vi "Configure Revert Worker.vi"() -> ()   [LabVIEW 2013, in "LVH-Revert.lvlib"]
uses:
  <vilib>/LabVIEW Hacker/Revert/LVH-Revert.lvlib
  <vilib>/Utility/config.llb/Read Key (String).vi
  <vilib>/Utility/config.llb/Read Key (Path).vi
  <vilib>/Utility/config.llb/Write Key (String).vi
  <vilib>/Utility/config.llb/Write Key (Path).vi
  <vilib>/Utility/config.llb/NI_LVConfig.lvlib
panel:
  in  "Archive Directory":path
  in  "Cancel Button":bool
  in  "Save Button":bool
  in  "Output Directory":path
  in  "Backsave Directory":path
  in  "Unzip Directory":path
  in  "Source Directory":path
  in  "Job Done Queue Name":string
  in  "Jobs Queue Name":string
  in  "AWS Account Number":string
  in  "AWS Secret Key":string
  in  "AWS Access Key ID":string
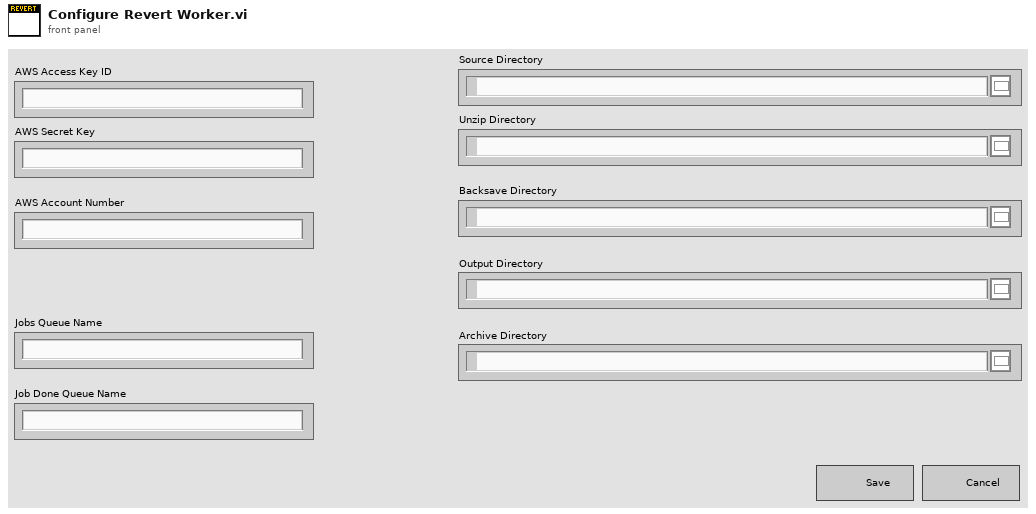
[diagram p1: front panel]
types:
  T1 = typedef "NI_LVConfig.lvlib/Config Data RefNum.ctl" = refnum<k1>
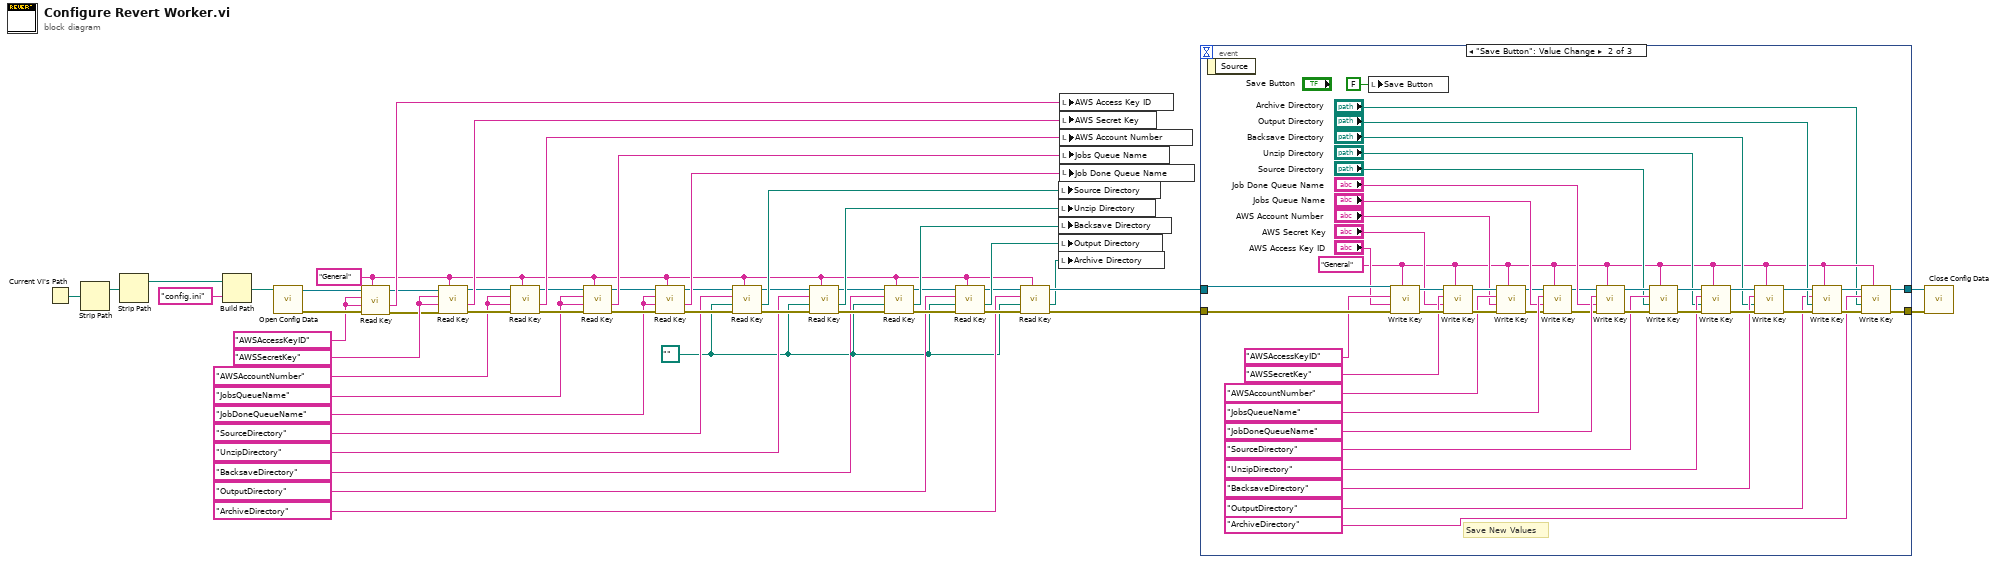
[diagram p0: block diagram]
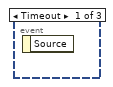
[diagram p2: hidden frame]
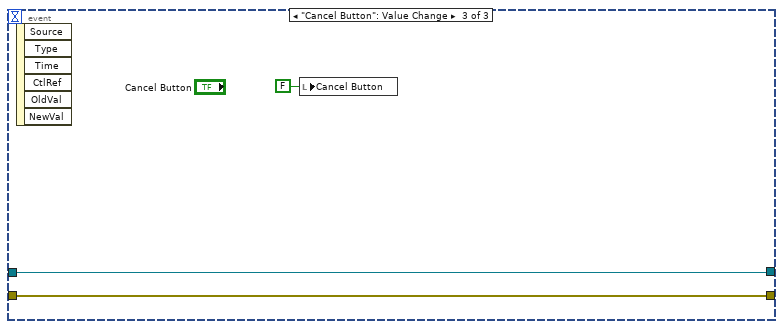
[diagram p3: hidden frame]
diagram:
  w2 = path "" ("Unzip Directory")
  w30 = "JobDoneQueueName"
  w32 = "JobsQueueName"
  w34 = "AWSAccountNumber"
  w36 = "AWSSecretKey"
  w38 = "AWSAccessKeyID"
  w4 = "General" ("section")
  n1 = Current VI's Path() -> (path=w51:path)
  n2 = Strip Path(path=w51) -> (stripped path=w50:path)  [unwired: 1 out]
  n3 = Strip Path(path=w50) -> (stripped path=w49:path)  [unwired: 1 out]
  n4 = Build Path(base path=w49, name or relative path="config.ini") -> (appended path=w47:path)
  n5 = call <vilib>:"Open Config Data.vi"("configuration file path"=w47) -> ("error out"=w46:errorcluster, "refnum"=w13:T1)  [unwired: 8 in, 1 out]
  n6 = call-poly <vilib>:"Read Key.vi"("section"=w4, "error in (no error)"=w46, "default value"=w38, "key"=w38, "refnum"=w13) -> ("error out"=w14:errorcluster, "value"=w37:string, "refnum out"=w12:T1)  [unwired: 3 in, 1 out]
  n7 = call-poly <vilib>:"Read Key.vi"("section"=w4, "error in (no error)"=w14, "default value"=w36, "key"=w36, "refnum"=w12) -> ("error out"=w45:errorcluster, "value"=w35:string, "refnum out"=w21:T1)  [unwired: 3 in, 1 out]
  n8 = call-poly <vilib>:"Read Key.vi"("section"=w4, "error in (no error)"=w45, "default value"=w34, "key"=w34, "refnum"=w21) -> ("error out"=w44:errorcluster, "value"=w33:string, "refnum out"=w20:T1)  [unwired: 3 in, 1 out]
  n9 = call-poly <vilib>:"Read Key.vi"("section"=w4, "error in (no error)"=w44, "default value"=w32, "key"=w32, "refnum"=w20) -> ("error out"=w43:errorcluster, "value"=w31:string, "refnum out"=w19:T1)  [unwired: 3 in, 1 out]
  n10 = call-poly <vilib>:"Read Key.vi"("section"=w4, "error in (no error)"=w43, "default value"=w30, "key"=w30, "refnum"=w19) -> ("error out"=w42:errorcluster, "value"=w29:string, "refnum out"=w18:T1)  [unwired: 3 in, 1 out]
  n11 = call-poly <vilib>:"Read Key.vi"("section"=w4, "error in (no error)"=w42, "default value"=w2, "key"="SourceDirectory", "refnum"=w18) -> ("error out"=w41:errorcluster, "value"=w27:path, "refnum out"=w17:T1)  [unwired: 3 in, 1 out]
  n12 = call-poly <vilib>:"Read Key.vi"("section"=w4, "error in (no error)"=w41, "default value"=w2, "key"="UnzipDirectory", "refnum"=w17) -> ("error out"=w40:errorcluster, "value"=w25:path, "refnum out"=w16:T1)  [unwired: 3 in, 1 out]
  n13 = call-poly <vilib>:"Read Key.vi"("section"=w4, "error in (no error)"=w40, "default value"=w2, "key"="BacksaveDirectory", "refnum"=w16) -> ("error out"=w39:errorcluster, "value"=w23:path, "refnum out"=w15:T1)  [unwired: 3 in, 1 out]
  n14 = call-poly <vilib>:"Read Key.vi"("section"=w4, "error in (no error)"=w39, "default value"=w2, "key"="OutputDirectory", "refnum"=w15) -> ("error out"=w8:errorcluster, "value"=w22:path, "refnum out"=w6:T1)  [unwired: 3 in, 1 out]
  n15 = call-poly <vilib>:"Read Key.vi"("section"=w4, "error in (no error)"=w8, "default value"=w2, "key"="ArchiveDirectory", "refnum"=w6) -> ("error out"=w7:errorcluster, "value"=w1:path, "refnum out"=w5:T1)  [unwired: 3 in, 1 out]
  n16 = local write "Source Directory"(w27) -> ()
  n17 = local write "Unzip Directory"(w25) -> ()
  n18 = local write "Backsave Directory"(w23) -> ()
  n19 = local write "Output Directory"(w22) -> ()
  n20 = local write "Archive Directory"(w1) -> ()
  n21 = local write "AWS Access Key ID"(w37) -> ()
  n22 = local write "AWS Secret Key"(w35) -> ()
  n23 = local write "AWS Account Number"(w33) -> ()
  n24 = local write "Jobs Queue Name"(w31) -> ()
  n25 = local write "Job Done Queue Name"(w29) -> ()
  n26 = event shown="[1] \"Save Button\": Value Change" {
    selector: _ -> [_ _ _]
    dyn-events: _ -> [_ _ _]
    timeout: _ -> [_ _ _]
    tunnel: w7 -> [_ w94 w97]
    tunnel: w5 -> [_ w93 w96]
    tunnel: [_ w55 w97] -> w10
    tunnel: [_ w56 w96] -> w9
    event Timeout {
      n27 = event-data() -> ()  [unwired: 1 in, 1 out]
    }
    event "Save Button": Value Change {
      w54 = "General" ("section")
      # "Save New Values"
      n28 = event-data() -> ()  [unwired: 1 in, 1 out]
      n29 = local write "Save Button"(FALSE ("Save Button")) -> ()
      n30 = call-poly <vilib>:"Write Key.vi"("section"=w54, "error in (no error)"=w94, "value"="AWS Access Key ID", "key"="AWSAccessKeyID", "refnum"=w93) -> ("error out"=w90:errorcluster, "refnum out"=w89:T1)  [unwired: 4 in, 1 out]
      n31 = call-poly <vilib>:"Write Key.vi"("section"=w54, "error in (no error)"=w90, "value"="AWS Secret Key", "key"="AWSSecretKey", "refnum"=w89) -> ("error out"=w86:errorcluster, "refnum out"=w85:T1)  [unwired: 4 in, 1 out]
      n32 = call-poly <vilib>:"Write Key.vi"("section"=w54, "error in (no error)"=w86, "value"="AWS Account Number", "key"="AWSAccountNumber", "refnum"=w85) -> ("error out"=w71:errorcluster, "refnum out"=w60:T1)  [unwired: 4 in, 1 out]
      n33 = call-poly <vilib>:"Write Key.vi"("section"=w54, "error in (no error)"=w71, "value"="Jobs Queue Name", "key"="JobsQueueName", "refnum"=w60) -> ("error out"=w70:errorcluster, "refnum out"=w59:T1)  [unwired: 4 in, 1 out]
      n34 = call-poly <vilib>:"Write Key.vi"("section"=w54, "error in (no error)"=w70, "value"="Job Done Queue Name", "key"="JobDoneQueueName", "refnum"=w59) -> ("error out"=w84:errorcluster, "refnum out"=w79:T1)  [unwired: 4 in, 1 out]
      n35 = call-poly <vilib>:"Write Key.vi"("section"=w54, "error in (no error)"=w84, "value"="Source Directory", "key"="SourceDirectory", "refnum"=w79) -> ("error out"=w83:errorcluster, "refnum out"=w80:T1)  [unwired: 4 in, 1 out]
      n36 = call-poly <vilib>:"Write Key.vi"("section"=w54, "error in (no error)"=w83, "value"="Unzip Directory", "key"="UnzipDirectory", "refnum"=w80) -> ("error out"=w82:errorcluster, "refnum out"=w81:T1)  [unwired: 4 in, 1 out]
      n37 = call-poly <vilib>:"Write Key.vi"("section"=w54, "error in (no error)"=w82, "value"="Backsave Directory", "key"="BacksaveDirectory", "refnum"=w81) -> ("error out"=w64:errorcluster, "refnum out"=w63:T1)  [unwired: 4 in, 1 out]
      n38 = call-poly <vilib>:"Write Key.vi"("section"=w54, "error in (no error)"=w64, "value"="Output Directory", "key"="OutputDirectory", "refnum"=w63) -> ("error out"=w58:errorcluster, "refnum out"=w57:T1)  [unwired: 4 in, 1 out]
      n39 = call-poly <vilib>:"Write Key.vi"("section"=w54, "error in (no error)"=w58, "value"="Archive Directory", "key"="ArchiveDirectory", "refnum"=w57) -> ("error out"=w55:errorcluster, "refnum out"=w56:T1)  [unwired: 4 in, 1 out]
    }
    event "Cancel Button": Value Change {
      n40 = event-data() -> ()  [unwired: 1 in, 6 out]
      n41 = local write "Cancel Button"(FALSE ("Cancel Button")) -> ()
    }
  }
  n42 = call <vilib>:"Close Config Data.vi"("error in (no error)"=w10, "refnum"=w9) -> ()  [unwired: 8 in, 2 out]
